vi "get_all_input_names.vi"(8 "error in (no error)":errorcluster, 11 "VISA resource name":refnum<visa-resource-name>) -> (0 "error out":errorcluster, 2 "Input names":string[](array[string]), 3 "VISA resource name out":refnum<visa-resource-name>)   [LabVIEW 2018]
doc: "Update all input names."
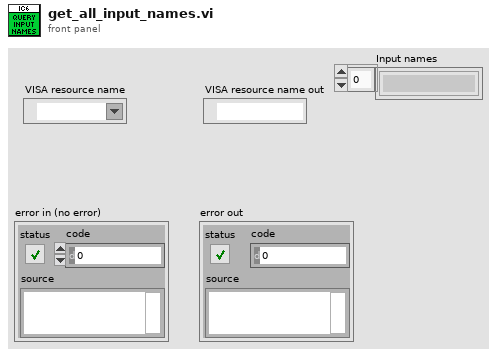
[diagram p1: front panel]
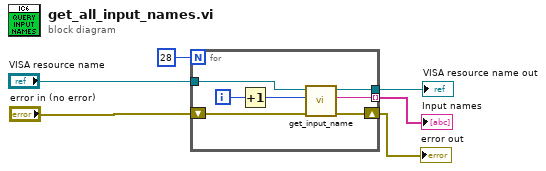
[diagram p0: block diagram]
diagram:
  n1 = for {
    N: 28 -> [_]
    shift-right: [w10] -> w6
    shift-left: "error in (no error)" -> [w11]
    tunnel: [w9] -> w4
    tunnel: [w8] -> w2 mode=indexing
    tunnel: "VISA resource name" -> [w7]
    i -> [w13]
    n2 = Increment(x=w13) -> (x+1=w12:i32)
    n3 = call "get_input_name.vi"("error in (no error)"=w11, "input number"=w12, "VISA resource name"=w7) -> ("error out"=w10:errorcluster, "input name"=w8:string, "VISA resource name out"=w9:refnum<visa-resource-name>)  [unwired: 6 in]
  }
  "error out" <- w6
  "VISA resource name out" <- w4
  "Input names" <- w2
